vi "TurnOff.vi"(8 "error in (no error)":errorcluster, 11 "PSU_N87 in":refnum<class "PSU_N87.lvclass">) -> (0 "error out":errorcluster, 3 "PSU_N87 out":refnum<class "PSU_N87.lvclass">)   [LabVIEW 2014, in "PSU_N87.lvclass"]
uses:
  PSU_N87.lvclass
  PSU_N87.lvclass/PSU_N87.ctl
  PSU.lvclass
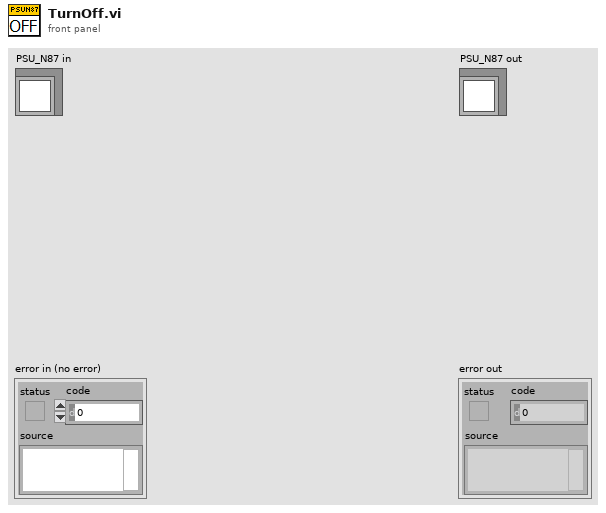
[diagram p1: front panel]
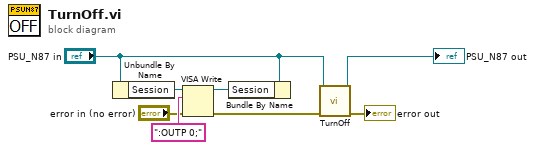
[diagram p0: block diagram]
diagram:
  n1 = Unbundle By Name("PSU_N87 in") -> ("Session"=w7:refnum<visa-resource-name>)
  n2 = VISA Write(VISA resource name=w7, write buffer=":OUTP 0;", error in (no error)="error in (no error)") -> (VISA resource name out=w5:refnum<visa-resource-name>, error out=w2:errorcluster)  [unwired: 1 out]
  n3 = Bundle By Name(cluster="PSU_N87 in", "Session"=w5) -> ()  [unwired: 1 out]
  n4 = call-parent "TurnOff.vi"("error in (no error)"=w2, "PSU in"="PSU_N87 in") -> ("error out"=→"error out":errorcluster, "PSU out"=→"PSU_N87 out":refnum<class "PSU_N87.lvclass">)  [unwired: 8 in]
